vi "DUAL GAUGE-RW Keyboard test.vi"(8 "Fehler (Eingang)":errorcluster, 11 "Referenz in":refnum<visa-resource-name>) -> (0 "Cluster (Ausgang)":errorcluster, 1 "Key 3":i32(ring) items=["Not pushed", "pushed"], 2 "Key 2":i32(ring) items=["Not pushed", "pushed"], 3 "Referenz out":refnum<visa-resource-name>, 4 "Key 4":i32(ring) items=["Not pushed", "pushed"], 5 "Key 1":i32(ring) items=["Not pushed", "pushed"])   [LabVIEW 2010, in "Dual Gauge.lvlib"]
uses:
  Dual Gauge.lvlib
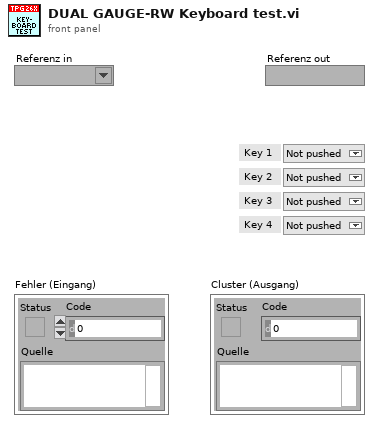
[diagram p1: front panel]
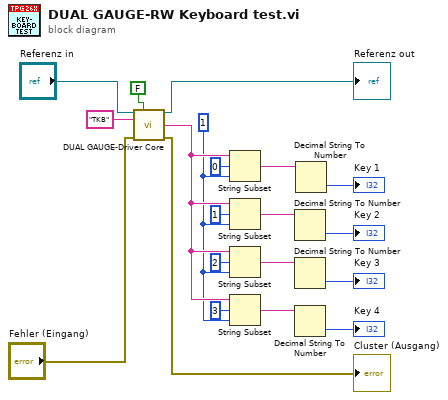
[diagram p0: block diagram]
diagram:
  w14 = 1 ("Länge")
  n1 = call "DUAL GAUGE-Driver Core.vi"("Referenz in"="Referenz in", "Write/Read"=FALSE ("W/R"), "Command"="TKB", "Fehler (Eingang)"="Fehler (Eingang)") -> ("Referenz out"=→"Referenz out":refnum<visa-resource-name>, "String Out"=w15:string, "Cluster (Ausgang)"=→"Cluster (Ausgang)":errorcluster)  [unwired: 9 in]
  n2 = String Subset(string=w15, offset (0)=0 ("Offset (0)"), length (rest)=w14) -> (substring=w9:string)
  n3 = String Subset(string=w15, offset (0)=1 ("Offset (0)"), length (rest)=w14) -> (substring=w8:string)
  n4 = String Subset(string=w15, offset (0)=2 ("Offset (0)"), length (rest)=w14) -> (substring=w7:string)
  n5 = String Subset(string=w15, offset (0)=3 ("Offset (0)"), length (rest)=w14) -> (substring=w6:string)
  n6 = Decimal String To Number(string=w8) -> (number=→"Key 2":i32)  [unwired: 2 in, 1 out]
  n7 = Decimal String To Number(string=w7) -> (number=→"Key 3":i32)  [unwired: 2 in, 1 out]
  n8 = Decimal String To Number(string=w6) -> (number=→"Key 4":i32)  [unwired: 2 in, 1 out]
  n9 = Decimal String To Number(string=w9) -> (number=→"Key 1":i32)  [unwired: 2 in, 1 out]
